vi "Measure Impedance R&S ZVL.vi"() -> ()   [LabVIEW 2016]
uses:
  Flow Control/Impedance Analyzer States.ctl
  Flow Control/Set_Read_Clear.ctl
  Save Trace/Global Variable Control.ctl
panel:
  out "Running":bool=TRUE
  in  "Tab Control 2":enum32{"Main", "Settings", "Scale"}(tab)
  out "Result File Path":path
  in  "Save":bool
  out "Result File Name":string
  in  "Frequency Range [Hz]":enum32{"Setting", "Actual"}(tab)
  in  "Frequency Range":T1={"Start [Hz]"=100000.0, "No. of points"=1600, "Stop [Hz]"=20000000.0} {"Stop [Hz]" format="%#_6p"; "Start [Hz]" format="%#_6p"}
  out "Frequency span":T2 {"Stop [Hz]" format="%#_6p"; "df [Hz]" format="%#_6p"; "Start [Hz]" format="%#_6p"}
  in  "Max. Update Rate [1/s]":dbl=10.0 min=0.1
  in  "R&S ZVL VISA Address":refnum<visa-resource-name>="ZVL13-100935"
  out "Error Out":errorcluster
  in  "Ref. Z [Ohm]":cdb=50.0+0.0i
  in  "File Prefix":string="ZVL_S11"
  in  "Extension":string="trc"
  in  "Channel":i32=1 min=1 max=2 step=1
  out "Actual Update Rate [1/s]":dbl
  in  "Frequency Axis [Hz]":cluster{dbl, dbl}(slide)={20000000.0, 0.0} scale=0.0..40000000.0 scale format="%#_6p"
  in  "Stop":bool
  in  "Display Tab":T3(tab)
  in  "Tab Control 4":enum32{"Separate", "Together"}(tab)
  out "Mag":T4(graph)
  out "Phase":T4(graph)
  out "arg abs":T5(graph)
  out "Re Im":T5(graph)
  out "S11":T5(graph)
  out "Y":cdb[](graph)
  # "Impedance Measurement\nRohde & Schwarz ZVL Network Analyzer"
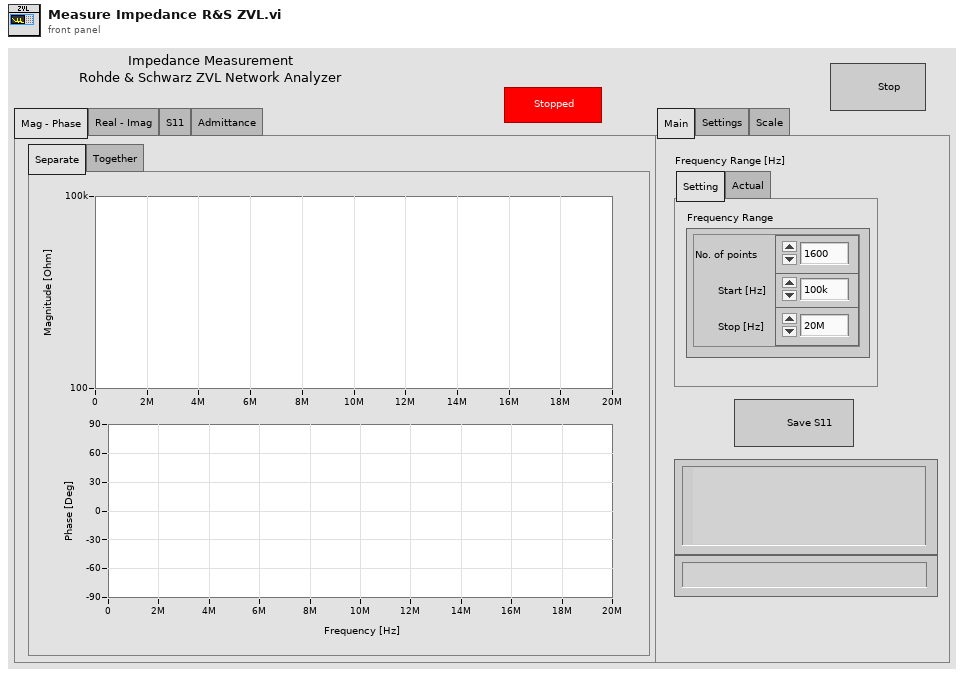
[diagram p1: front panel]
types:
  T1 = cluster{"Start [Hz]":dbl, "No. of points":i32, "Stop [Hz]":dbl}
  T2 = cluster{"Start [Hz]":dbl, "No. of points":i32, "df [Hz]":dbl, "Stop [Hz]":dbl}
  T3 = enum32{"Mag - Phase", "Real - Imag", "S11", "Admittance"}
  T4 = cluster{"f0 [Hz]":dbl, "df [Hz]":dbl, "Value":dbl[]}
  T5 = cluster{"f0 [Hz]":dbl, "df [Hz]":dbl, "Value":dbl[]}[]
  T6 = typedef "Set_Read_Clear.ctl" = enum16{"Clear", "Set", "Read"}
  T7 = typedef "Impedance Analyzer States.ctl" = enum16{"Save Calibration", "Recall Calibration", "Initialize", "Idle", "Save State", "Load State", "Setup Sequence", "Aquire Traces", "Display Result", "Save Result", "Shutdown", "Quit"}
  T8 = typedef "Global Variable Control.ctl" = enum16{"Clear", "Set", "Get"}
  T9 = enum16{"int8", "int16", "int32", "uint8", "uint16", "uint32", "float32", "float64", "complex64", "complex128"}
  T10 = typedef "Trace (cplx).ctl" = cluster{"x0":dbl, "dx":dbl, "Z":cdb[]}
  T11 = typedef "Trace (dbl).ctl" = cluster{"x0 ":dbl, "dx":dbl, "Y":dbl[]}
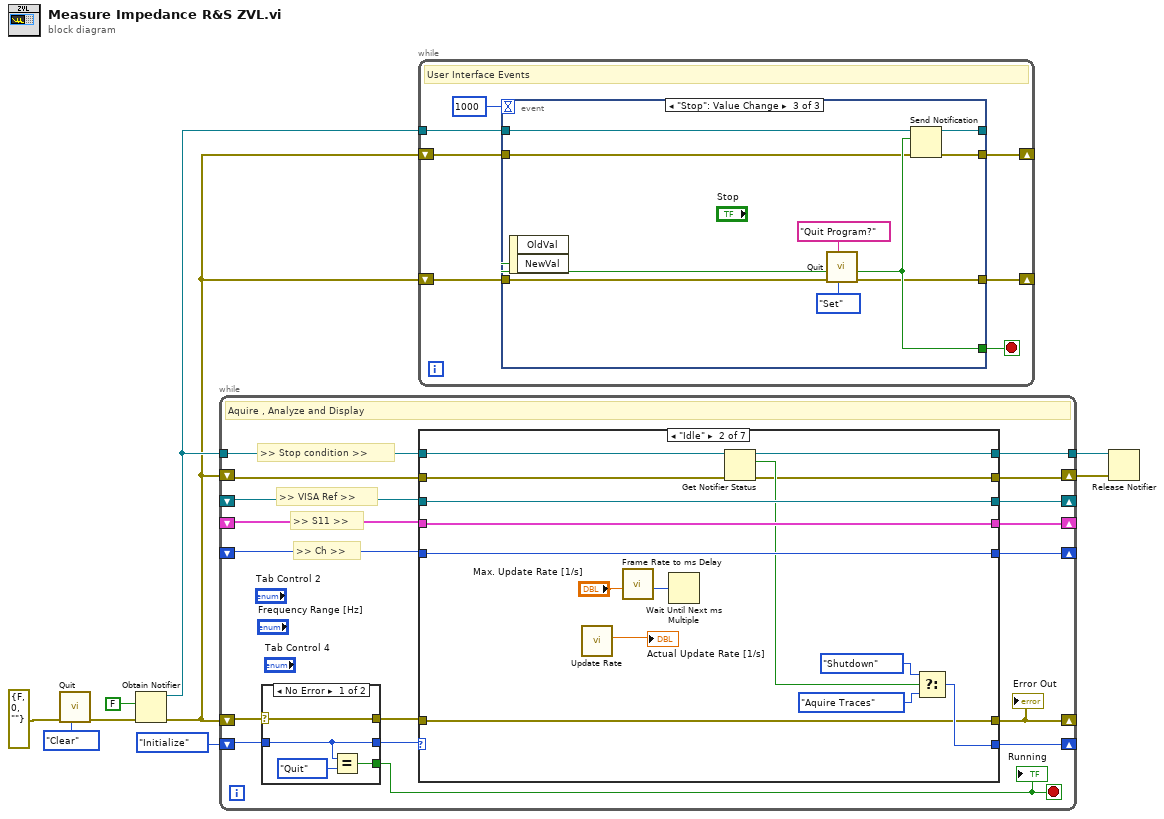
[diagram p0: block diagram]
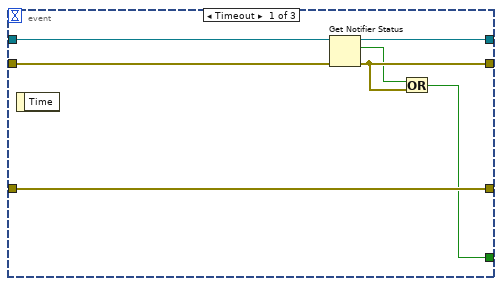
[diagram p2: hidden frame]
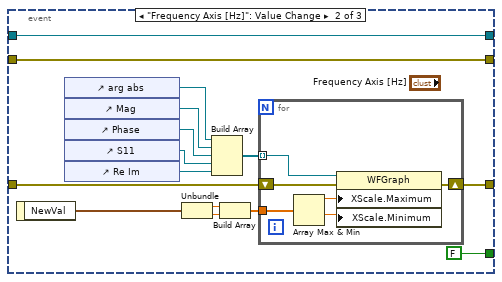
[diagram p3: hidden frame]
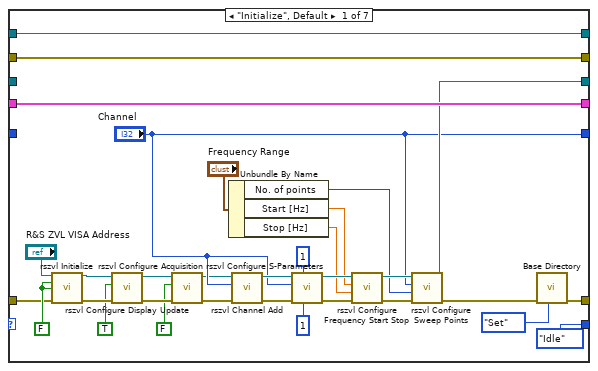
[diagram p4: hidden frame]
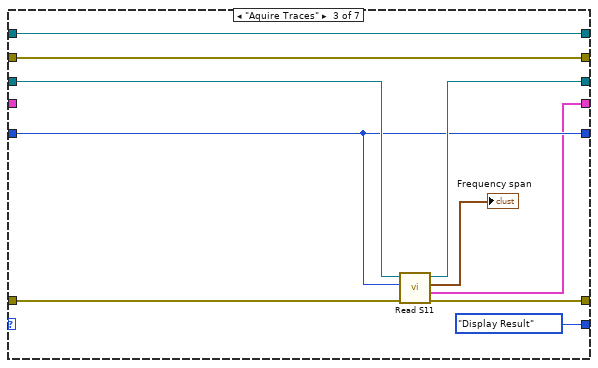
[diagram p5: hidden frame]
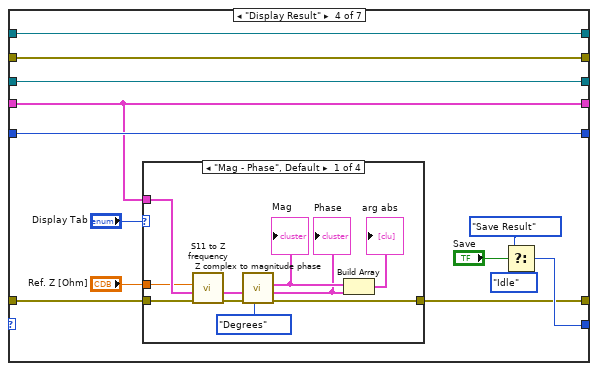
[diagram p6: hidden frame]
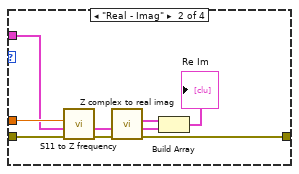
[diagram p7: hidden frame]
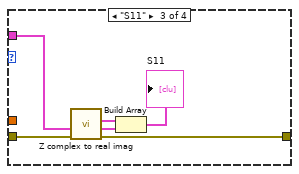
[diagram p8: hidden frame]
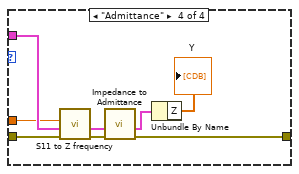
[diagram p9: hidden frame]
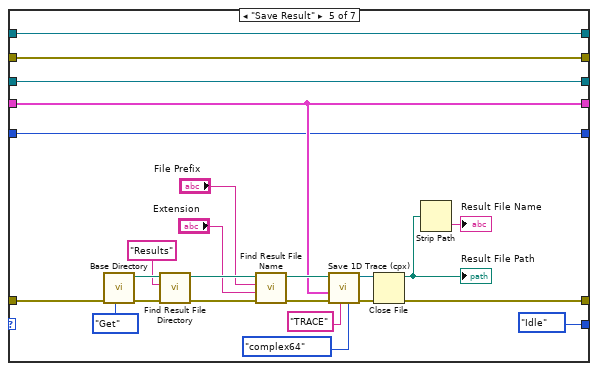
[diagram p10: hidden frame]
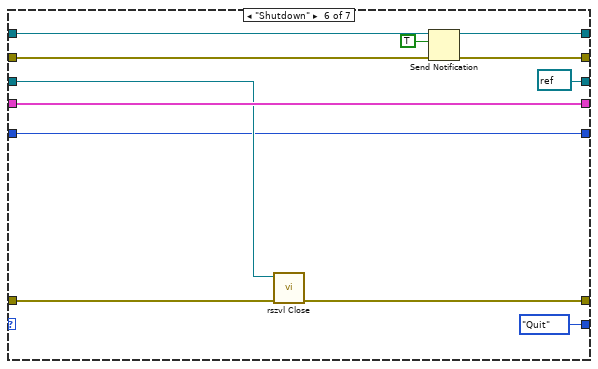
[diagram p11: hidden frame]
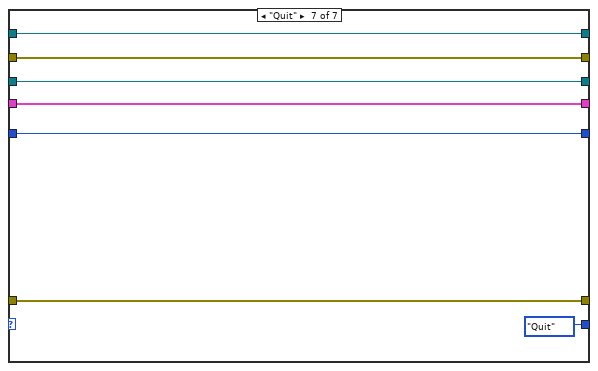
[diagram p12: hidden frame]
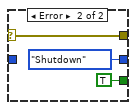
[diagram p13: hidden frame]
diagram:
  n1 = call "Quit.vi"("Operation"=Set_Read_Clear."Clear", "Error In"=errorcluster {"status"=FALSE, "code"=0, "source"=""} ("error out")) -> ("Error Out"=w5:errorcluster)  [unwired: 8 in, 1 out]
  n2 = Obtain Notifier(notification data type=FALSE, error in (no error)=w5) -> (notifier out=w6:refnum<notifier>, error out=w2:errorcluster)  [unwired: 2 in, 1 out]
  n3 = while {
    shift-right: [w23] -> _
    shift-left: w2 -> [w17]
    shift-right: [w26] -> _
    shift-left: Impedance_Analyzer_States."Initialize" -> [w15]
    shift-right: [w25] -> _
    shift-left: _ -> [w24]
    shift-right: [w22] -> _
    shift-left: _ -> [w21]
    shift-right: [w19] -> _
    shift-left: _ -> [w20]
    tunnel: w6 -> [w13]
    tunnel: [w12] -> w3
    shift-right: [w11] -> w1
    shift-left: w2 -> [w10]
    stop <- w14 stop-if-true
    # ">> Stop condition >>"
    # ">> Ch >>"
    # ">> S11 >>"
    # ">> VISA Ref >>"
    # "Aquire , Analyze and Display"
    n4 = case shown="No Error" w17 {
      selector: w17 -> [w172 w177]
      tunnel: [w173 Impedance_Analyzer_States."Shutdown" ("y")] -> w18
      tunnel: [w172 w177] -> w16
      tunnel: w15 -> [w173 _]
      tunnel: [w174 TRUE] -> w14
      frame No Error {
        n5 = Equal?(x=w173, y=Impedance_Analyzer_States."Quit") -> (x = y?=w174:bool)
      }
      frame Error {
      }
    }
    "Running" <- w14
    n6 = case shown="\"Idle\"" w18 {
      tunnel: [w57 w60 w76 w89 w137 w156 w170] -> w23
      tunnel: w16 -> [w52 w60 w81 w90 w143 w160 w170]
      tunnel: [Impedance_Analyzer_States."Idle" w66 Impedance_Analyzer_States."Display Result" w92 Impedance_Analyzer_States."Idle" Impedance_Analyzer_States."Quit" Impedance_Analyzer_States."Quit"] -> w26
      tunnel: [w43 w73 w79 w96 w153 refnum<visa-resource-name> refnum ("VISA resource name out") w171] -> w25
      tunnel: w24 -> [_ w73 w82 w96 w153 w161 w171]
      tunnel: [w55 w72 w77 w87 w141 w162 w168] -> w22
      tunnel: w21 -> [w55 w72 _ w87 w141 w162 w168]
      tunnel: w20 -> [_ w71 w78 w95 w132 w159 w167]
      tunnel: ["Channel" w71 w78 w95 w132 w159 w167] -> w19
      tunnel: w13 -> [w36 w64 w75 w85 w131 w157 w166]
      tunnel: [w36 w63 w75 w85 w131 w157 w166] -> w12
      tunnel: [w35 w62 w74 w84 w130 w154 w165] -> w11
      tunnel: w10 -> [w35 w61 w74 w84 w130 w155 w165]
      frame "Initialize", Default {
        w53 = FALSE
        n7 = call <instrlib>:"rszvl Initialize.vi"("VISA resource name"="R&S ZVL VISA Address", "ID Query (Check)"=w53, "Reset (Reset)"=w53, "error in (no error)"=w52) -> ("VISA resource name out"=w38:refnum<visa-resource-name>, "error out"=w39:errorcluster)  [unwired: 10 in]
        n8 = call <instrlib>:"rszvl Configure Display Update.vi"("error in (no error)"=w39, "Display Update (Off)"=TRUE, "VISA resource name"=w38) -> ("error out"=w30:errorcluster, "VISA resource name out"=w31:refnum<visa-resource-name>)  [unwired: 7 in]
        n9 = call <instrlib>:"rszvl Configure Acquisition.vi"("error in (no error)"=w30, "Sweep Mode Continuous (On)"=FALSE, "VISA resource name"=w31) -> ("error out"=w29:errorcluster, "VISA resource name out"=w28:refnum<visa-resource-name>)  [unwired: 7 in]
        n10 = Unbundle By Name("Frequency Range") -> ("No. of points"=w42:i32, "Start [Hz]"=w45:dbl, "Stop [Hz]"=w44:dbl)
        n11 = call <instrlib>:"rszvl Channel Add.vi"("error in (no error)"=w29, "Channel (1)"="Channel", "VISA resource name"=w28) -> ("error out"=w34:errorcluster, "VISA resource name out"=w33:refnum<visa-resource-name>)  [unwired: 7 in]
        n12 = call <instrlib>:"rszvl Configure S-Parameters.vi"("In Port (1)"=1, "Out Port (1)"=1, "error in (no error)"=w34, "Channel (1)"="Channel", "VISA resource name"=w33) -> ("error out"=w49:errorcluster, "VISA resource name out"=w51:refnum<visa-resource-name>)  [unwired: 5 in]
        n13 = call <instrlib>:"rszvl Configure Frequency Start Stop.vi"("error in (no error)"=w49, "Stop Frequency (3.0e+9)"=w44, "Start Frequency (0.0)"=w45, "VISA resource name"=w51) -> ("error out"=w48:errorcluster, "VISA resource name out"=w50:refnum<visa-resource-name>)  [unwired: 6 in]
        n14 = call <instrlib>:"rszvl Configure Sweep Points.vi"("error in (no error)"=w48, "Number Of Points (201)"=w42, "Channel (1)"="Channel", "VISA resource name"=w50) -> ("error out"=w47:errorcluster, "VISA resource name out"=w43:refnum<visa-resource-name>)  [unwired: 6 in]
        n15 = call "Base Directory.vi"("Operation"=Global_Variable_Control."Set", "Error In"=w47) -> ("Error Out"=w57:errorcluster)  [unwired: 8 in, 1 out]
      }
      frame "Idle" {
        n16 = call "Update Rate.vi"() -> ("Update Rate [1/s]"=→"Actual Update Rate [1/s]":dbl)  [unwired: 9 in, 2 out]
        n17 = call "Frame Rate to ms Delay.vi"("Update rate [1/s]"="Max. Update Rate [1/s]") -> ("Wait [ms"=w69:u32)  [unwired: 10 in]
        n18 = Wait Until Next ms Multiple(millisecond multiple=w69) -> ()  [unwired: 1 out]
        n19 = Get Notifier Status(notifier=w64, error in (no error)=w61) -> (notifier out=w63:refnum<notifier>, current notification=w65:bool, error out=w62:errorcluster)  [unwired: 2 out]
        n20 = Select(t=Impedance_Analyzer_States."Shutdown", s=w65, f=Impedance_Analyzer_States."Aquire Traces") -> (s? t:f=w66:T7)
      }
      frame "Aquire Traces" {
        n21 = call "Read S11.vi"("Error In"=w81, "Channel (1)"=w78, "VISA Refnum In"=w82) -> ("Error Out"=w76:errorcluster, "S11"=w77:T10, "Frequency span"=→"Frequency span":T2, "VISA Refnum Out"=w79:refnum<visa-resource-name>)  [unwired: 5 in]
      }
      frame "Display Result" {
        n22 = case shown="\"Mag - Phase\", Default" "Display Tab" {
          tunnel: w87 -> [w105 w112 w119 w128]
          tunnel: w90 -> [w106 w115 w118 w129]
          tunnel: [w100 w110 w117 w124] -> w89
          tunnel: "Ref. Z [Ohm]" -> [w104 w113 _ w127]
          frame "Mag - Phase", Default {
            n23 = call "S11 to Z frequency.vi"("Error In"=w106, "S11"=w105, "Ref. Z [Ohm]"=w104) -> ("Error Out"=w103:errorcluster, "Z"=w102:T10)  [unwired: 7 in]
            n24 = call "Z complex to magnitude phase.vi"("Angle unit"=enum16{"Radians", "Degrees"}."Degrees", "Error In"=w103, "Z (cplx)"=w102) -> ("Error Out"=w100:errorcluster, "arg Z"=w98:T11, "|Z|"=w99:T11)  [unwired: 6 in]
            "Mag" <- w99
            "Phase" <- w98
            n25 = Build Array(w99, w98) -> (→"arg abs":T11[])
          }
          frame "Real - Imag" {
            n26 = call "S11 to Z frequency.vi"("Error In"=w115, "S11"=w112, "Ref. Z [Ohm]"=w113) -> ("Error Out"=w114:errorcluster, "Z"=w111:T10)  [unwired: 7 in]
            n27 = call "Z complex to real imag.vi"("Error In"=w114, "Z (cplx)"=w111) -> ("Error Out"=w110:errorcluster, "imag Z"=w108:T11, "real Z"=w109:T11)  [unwired: 7 in]
            n28 = Build Array(w109, w108) -> (→"Re Im":T11[])
          }
          frame "S11" {
            n29 = call "Z complex to real imag.vi"("Error In"=w118, "Z (cplx)"=w119) -> ("Error Out"=w117:errorcluster, "imag Z"=w116:T11, "real Z"=w121:T11)  [unwired: 7 in]
            n30 = Build Array(w121, w116) -> (→"S11":T11[])
          }
          frame "Admittance" {
            n31 = call "S11 to Z frequency.vi"("Error In"=w129, "S11"=w128, "Ref. Z [Ohm]"=w127) -> ("Error Out"=w126:errorcluster, "Z"=w125:T10)  [unwired: 7 in]
            n32 = call "Impedance to Admittance.vi"("Error In"=w126, "Z (cplx)"=w125) -> ("Error Out"=w124:errorcluster, "Y (complex)"=w123:T10)  [unwired: 8 in]
            n33 = Unbundle By Name(w123) -> ("Z"=→"Y":cdb[])
          }
        }
        n34 = Select(t=Impedance_Analyzer_States."Save Result", s="Save", f=Impedance_Analyzer_States."Idle") -> (s? t:f=w92:T7)
      }
      frame "Save Result" {
        n35 = call "Base Directory.vi"("Operation"=Global_Variable_Control."Get", "Error In"=w143) -> ("Error Out"=w147:errorcluster, "Base Directory"=w145:path)  [unwired: 8 in]
        n36 = call "Find Result File Directory.vi"("error in (no error)"=w147, "Directory Name"="Results", "Parent Path"=w145) -> ("error out"=w150:errorcluster, "Result Directory"=w151:path)  [unwired: 7 in]
        n37 = call "Find Result File Name.vi"("Error In"=w150, "Extension"="Extension", "Prefix"="File Prefix", "Directory"=w151) -> ("error out"=w140:errorcluster, "Result File Path"=w142:path)  [unwired: 4 in, 2 out]
        n38 = call "Save 1D Trace (cpx).vi"("Data Type"=T9."complex64", "Contents ID"="TRACE", "Error In"=w140, "Trace"=w141, "File Path"=w142) -> ("Error Out"=w138:errorcluster, "File Refnum Out"=w139:refnum<file>)  [unwired: 5 in]
        n39 = Close File(refnum=w139, error in=w138) -> (path=w133:path, error out=w137:errorcluster)
        "Result File Path" <- w133
        n40 = Strip Path(path=w133) -> (name=→"Result File Name":string)  [unwired: 1 out]
      }
      frame "Shutdown" {
        n41 = call <instrlib>:"rszvl Close.vi"("error in (no error)"=w160, "VISA resource name"=w161) -> ("error out"=w156:errorcluster)  [unwired: 9 in]
        n42 = Send Notification(notification=TRUE ("Quit"), notifier=w157, error in (no error)=w155) -> (error out=w154:errorcluster)  [unwired: 1 out]
      }
      frame "Quit" {
      }
    }
    "Error Out" <- w23
  }
  n43 = while {
    shift-right: [w185] -> _
    shift-left: w2 -> [w184]
    tunnel: w6 -> [w182]
    shift-right: [w179] -> _
    shift-left: w2 -> [w180]
    stop <- w183 stop-if-true
    # "User Interface Events"
    n44 = event shown="[2] \"Stop\": Value Change" {
      selector: _ -> [_ _ _]
      dyn-events: _ -> [_ _ _]
      timeout: 1000 -> [_ _ _]
      tunnel: w184 -> [w189 w201 w221]
      tunnel: [w189 w200 w217] -> w185
      tunnel: [w186 FALSE ("Quit?") w218] -> w183
      tunnel: w182 -> [w192 w193 w219]
      tunnel: w180 -> [w190 w194 w216]
      tunnel: [w188 w194 w215] -> w179
      tunnel: [w191 w193 w214] -> _
      event Timeout {
        n45 = event-data() -> ()  [unwired: 1 in, 1 out]
        n46 = Get Notifier Status(notifier=w192, error in (no error)=w190) -> (notifier out=w191:refnum<notifier>, current notification=w187:bool, error out=w188:errorcluster)  [unwired: 2 out]
        n47 = Or(x=w187, y=w188) -> (x .or. y?=w186:bool)
      }
      event "Frequency Axis [Hz]": Value Change {
        n48 = event-data() -> ("NewVal"=w198:cluster{dbl, dbl})  [unwired: 1 in]
        n49 = control-ref of="arg abs"() -> (w207:refnum<vi>)
        n50 = control-ref of="Mag"() -> (w203:refnum<vi>)
        n51 = control-ref of="Phase"() -> (w206:refnum<vi>)
        n52 = control-ref of="S11"() -> (w202:refnum<vi>)
        n53 = control-ref of="Re Im"() -> (w205:refnum<vi>)
        n54 = Unbundle(w198) -> (w197:dbl, w196:dbl)
        n55 = Build Array(w207, w203, w206, w202, w205) -> (w204:refnum<vi>[])
        n56 = Build Array(w197, w196) -> (w195:dbl[])
        n57 = for {
          shift-right: [w212] -> w200
          shift-left: w201 -> [w213]
          tunnel: w204 -> [w211] mode=indexing
          tunnel: w195 -> [w208]
          n58 = Array Max & Min(array=w208) -> (max value=w210:dbl, min value=w209:dbl)  [unwired: 2 out]
          n59 = property class="WFGraph"(reference=w211, error in=w213, "XScale.Maximum"=w210, "XScale.Minimum"=w209) -> (error out=w212:errorcluster)  [unwired: 1 out]
        }
      }
      event "Stop": Value Change {
        n60 = event-data() -> ("NewVal"=w220:bool)  [unwired: 1 in, 1 out]
        n61 = call "Quit.vi"("Operation"=Set_Read_Clear."Set", "Message (Quit Program?)"="Quit Program?" ("message"), "Error In"=w221, "Quit"=w220) -> ("Error Out"=w217:errorcluster, "Quit?"=w218:bool)  [unwired: 6 in]
        n62 = Send Notification(notification=w218, notifier=w219, error in (no error)=w216) -> (notifier out=w214:refnum<notifier>, error out=w215:errorcluster)
      }
    }
  }
  n63 = Release Notifier(notifier=w3, error in (no error)=w1) -> ()  [unwired: 1 in, 3 out]
